vi "New Top Window Layout.vi"(8 "Error In":errorcluster, 9 "StatusBar (Toggable)":refnum<class "StatusBar.lvclass">, 10 "SideMenu (Toggable)":refnum<class "SideMenu.lvclass">, 11 "TitleBar (Toggable)":refnum<class "TitleBar.lvclass">) -> (0 "Error Out":errorcluster, 3 "Top Window Layout":refnum<class "Layout.lvclass">)   [LabVIEW 2021, in "Appearance Actor.lvlib" / "Top Window.lvclass"]
uses:
  Top Window.lvclass
  Layout/Layout.lvclass
  Layout Components/SideMenus/SideMenu/SideMenu.lvclass
  C:/Users/Thomas/Documents/Projects/TemplateVIEW/Sources/Appearance Actor/Layout Classes/Layout Components/Layout Component Class/Layout Component.lvclass
  Layout Components/StatusBars/StatusBar/StatusBar.lvclass
  Layout Components/TitleBars/TitleBar/TitleBar.lvclass
  C:/Users/Thomas/Documents/Projects/TemplateVIEW/Sources/Appearance Actor/Layout Classes/Layout/Layout.lvclass
  Layout/Layout.lvclass/Layout.ctl
  Layout/API/Data Member Access/Set TitleBar.vi
  Layout/API/Data Member Access/Set SideMenu.vi
  Layout/API/Data Member Access/Set StatusBar.vi
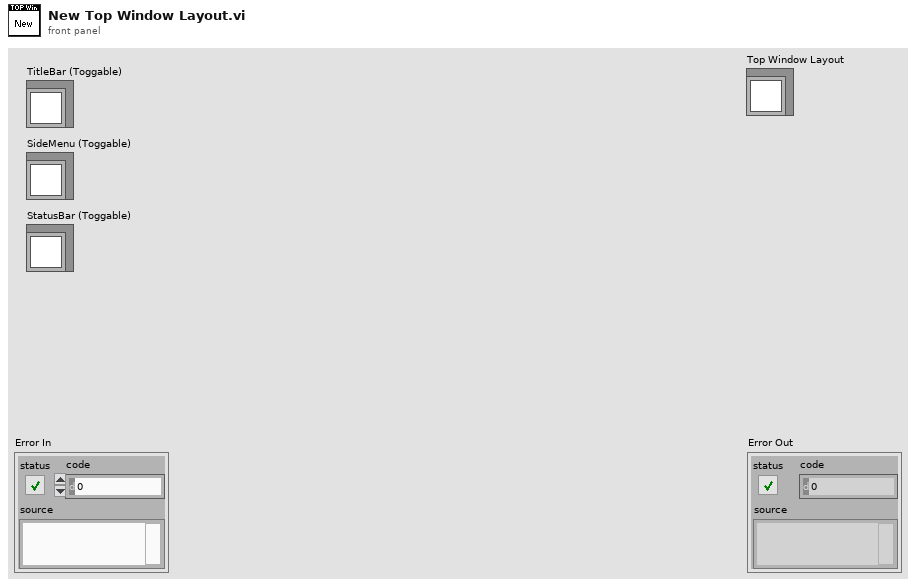
[diagram p1: front panel]
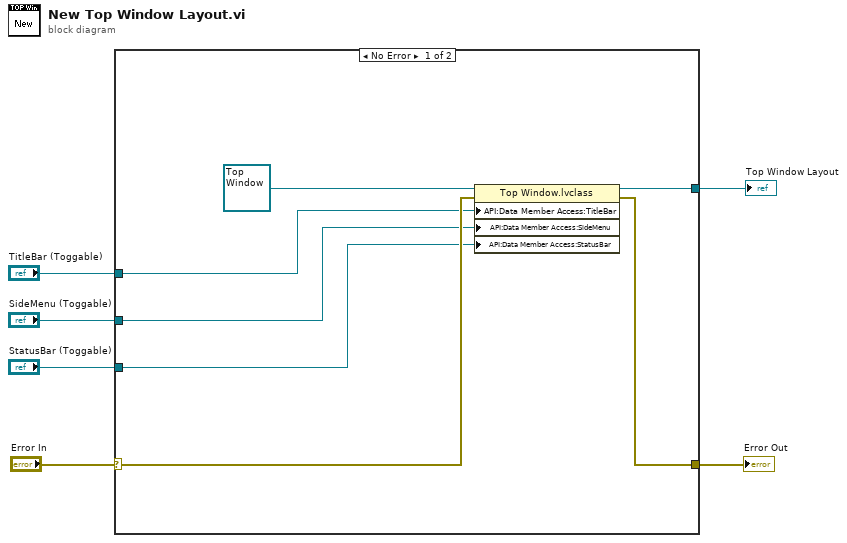
[diagram p0: block diagram]
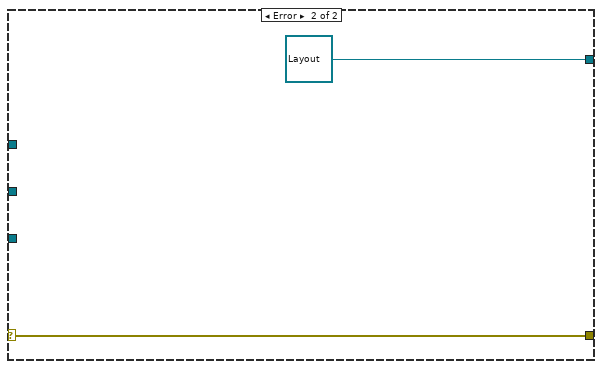
[diagram p2: hidden frame]
diagram:
  n1 = case shown="No Error" "Error In" {
    selector: "Error In" -> [w11 w15]
    tunnel: [w10 w15] -> w5
    tunnel: [w12 refnum<class "Layout.lvclass"> refnum ("Appearance Actor.lvlib:Layout.lvclass")] -> w4
    tunnel: "TitleBar (Toggable)" -> [w9 _]
    tunnel: "SideMenu (Toggable)" -> [w8 _]
    tunnel: "StatusBar (Toggable)" -> [w7 _]
    frame No Error {
      n2 = property class="Top Window.lvclass"(reference=refnum<class "Top Window.lvclass"> refnum ("Appearance Actor.lvlib:Top Window.lvclass"), error in=w11, "API:Data Member Access:TitleBar"=w9, "API:Data Member Access:SideMenu"=w8, "API:Data Member Access:StatusBar"=w7) -> (reference out=w12:refnum<class "Top Window.lvclass">, error out=w10:errorcluster)
    }
    frame Error {
    }
  }
  "Error Out" <- w5
  "Top Window Layout" <- w4
